vi "POST_receiveNew_ServoStatus_fromClient.vi"(3 "LabVIEW Web Service Request":refnum<class "Web Request.lvclass">) -> (1 "response":string)   [LabVIEW 2024]
uses:
  <vilib>/wsapi/Web Request.lvclass
panel:
  out "Status From Client":cluster{"mode":string, "position":dbl}
  # "Use the Web Service Request input terminal to call the VIs on the Web Services palette. Do not remove it from the connector pane unless you don't need access to the palette."
  # "Each additional control wired to the connector pane will be available as an input in the URL. To include an indicator in terminal-mode output (the default setting), it must also be wired to the connector pane."
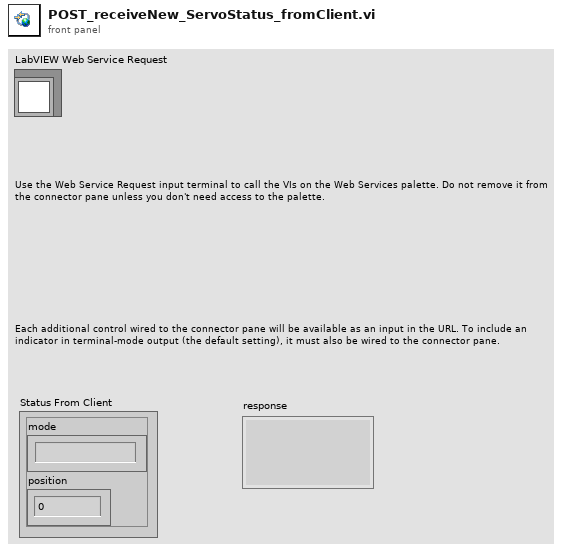
[diagram p1: front panel]
types:
  T1 = cluster{"status":cluster{"mode":string, "position":i16}}
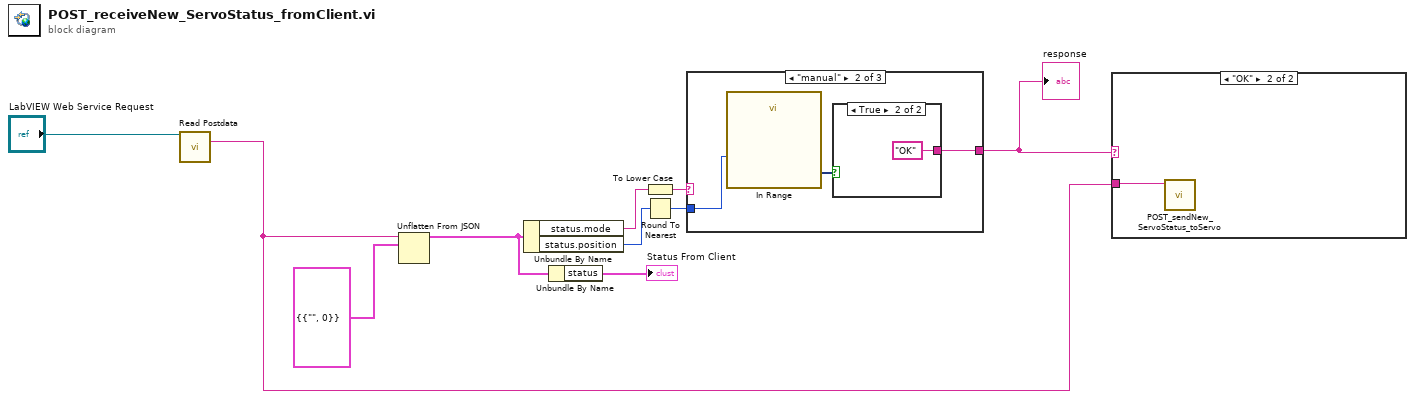
[diagram p0: block diagram]
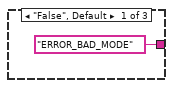
[diagram p3: hidden frame]
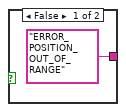
[diagram p4: hidden frame]
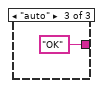
[diagram p5: hidden frame]
diagram:
  n1 = call <vilib>:"Read Postdata.vi"("LabVIEW Web Service Request"="LabVIEW Web Service Request") -> ("postdata"=w1:string)  [unwired: 12 in, 2 out]
  n2 = Unflatten From JSON(JSON string=w1, type and defaults=T1 {"status"={"mode"="", "position"=0}}) -> (value=w4:T1)  [unwired: 5 in, 1 out]
  n3 = Unbundle By Name "Unbundle By Name"(w4) -> ("status.mode"=w8:string, "status.position"=w9:i16)
  n4 = Unbundle By Name(w4) -> ("status"=→"Status From Client":cluster{"mode":string, "position":i16})
  n5 = To Lower Case(string=w8) -> (all lower case string=w7:string)
  n6 = Round To Nearest(number=w9) -> (nearest integer value=w6:i16)
  n7 = case shown="\"manual\"" w7 {
    tunnel: w6 -> [_ w12 _]
    tunnel: ["ERROR_BAD_MODE" w13 "OK"] -> w2
    frame "False", Default {
    }
    frame "manual" {
      n8 = call "In Range"("Operand 1"=w12) -> ("Result"=w14:dynamicdata)  [unwired: 9 in, 1 out]
      n9 = case shown="True" w14 {
        tunnel: ["ERROR_POSITION_OUT_OF_RANGE" "OK"] -> w13
        frame False {
        }
        frame True {
        }
      }
    }
    frame "auto" {
    }
  }
  "response" <- w2
  n10 = case shown="\"OK\"" w2 {
    tunnel: w1 -> [_ w18]
    frame Default {
    }
    frame "OK" {
      n11 = call "POST_sendNew_ServoStatus_toServo.vi"("JSON_ServoStatus_fromClient"=w18) -> ()  [unwired: 9 in, 2 out]
    }
  }
